vi "PAQmem_FindStartStopTimeIndex.vi"(8 "error in (no error)":errorcluster, 9 "End-time":timestamp, 10 "Start-time":timestamp, 11 "PAQ-memory in":refnum<class "PAQ-memory.lvclass">) -> (0 "error out":errorcluster, 1 "Size":i32, 2 "Start":i32, 3 "PAQ-memory out":refnum<class "PAQ-memory.lvclass">, 4 "time":timestamp[](array[timestamp]))   [LabVIEW 2020, in "Sgraph_lib_V1.lvlib" / "PAQ-memory.lvclass"]
doc: "Andre Koelewijn, 2 April 2021\n\nFind the index of the start and stop time when searching for a portion of the PAQ buffer section\nAdditional to the indexes this vi also delivers the time array of the searched data portion."
uses:
  PAQ-memory.lvclass
  PAQ-memory.lvclass/PAQ-memory.ctl
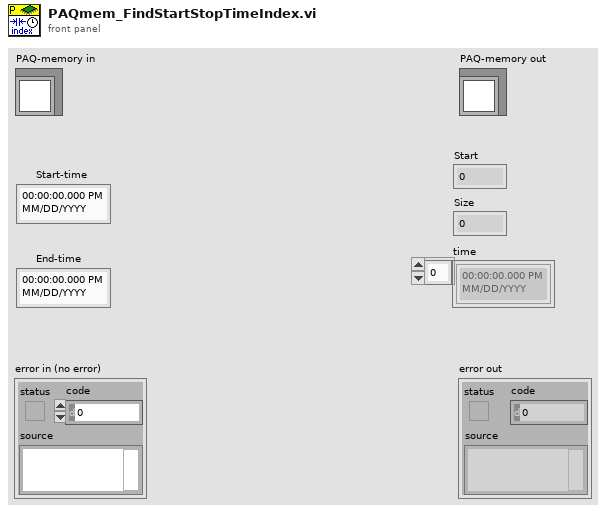
[diagram p1: front panel]
types:
  T1 = typedef "Sgraph_lib_V1.lvlib/FAMM.lvclass/typedef_PAQdata.ctl" = cluster{"TAGs":string[], "Time":refnum<data-value>, "TAGdata":cluster{"source":refnum<data-value>, "status":refnum<data-value>, "data":refnum<data-value>, "max":refnum<data-value>, "min":refnum<data-value>}[]}
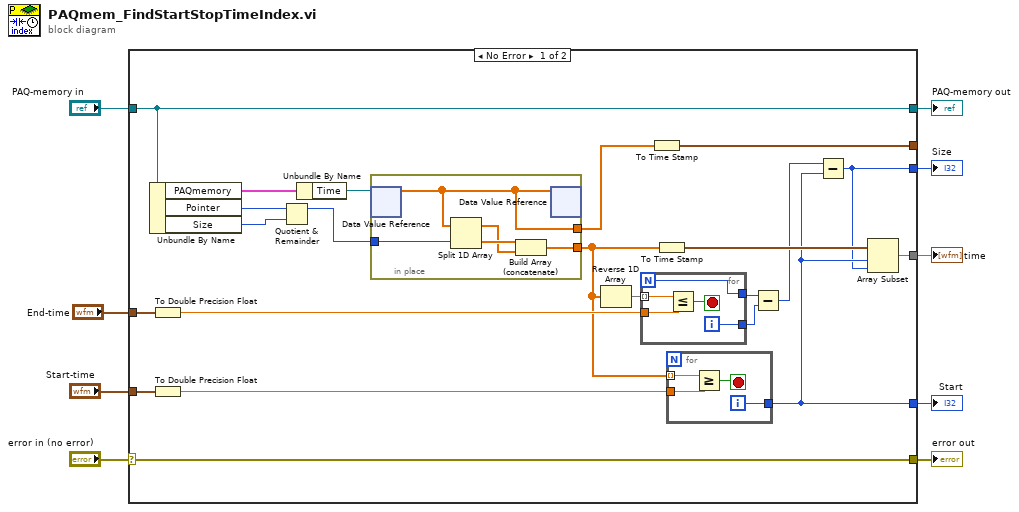
[diagram p0: block diagram]
diagram:
  n1 = case shown="No Error" "error in (no error)" {
    selector: "error in (no error)" -> [w31 w47]
    tunnel: [w31 w47] -> w8
    tunnel: [w29 w46] -> w6
    tunnel: "PAQ-memory in" -> [w29 w46]
    tunnel: [w23 _] -> w2
    tunnel: "Start-time" -> [w26 _]
    tunnel: [w19 _] -> w4
    tunnel: [w18 _] -> w3
    tunnel: "End-time" -> [w21 _]
    tunnel: [w10 _] -> _
    frame No Error {
      n2 = Unbundle By Name(w29) -> ("PAQmemory"=w30:T1, "Pointer"=w27:i32, "Size"=w22:i32)
      n3 = To Double Precision Float(number=w21) -> (double precision float=w20:dbl)
      n4 = To Double Precision Float(number=w26) -> (double precision float=w25:dbl)
      n5 = Quotient & Remainder(x=w27, y=w22) -> (x-y*floor(x/y)=w28:i32)  [unwired: 1 out]
      n6 = Unbundle By Name(w30) -> ("Time"=w12:refnum<data-value>)
      n7 = in-place {
        in-place-border: w28 -> [w45]
        in-place-border: [w42] -> w17
        in-place-border: [w41] -> w11
        n8 = in-place-dvr #1(w12) -> (w41:dbl[])  [unwired: 1 out]
        n9 = Split 1D Array(array=w41, index=w45) -> (first subarray=w43:dbl[], second subarray=w44:dbl[])
        n10 = Build Array (concatenate)(w44, w43) -> (w42:dbl[])
        n11 = in-place-dvr #1(w41) -> ()  [unwired: 2 out]
      }
      n12 = Reverse 1D Array(array=w17) -> (reversed array=w16:dbl[])
      n13 = for {
        N -> [w32]
        tunnel: w16 -> [w36] mode=indexing
        tunnel: w20 -> [w35]
        tunnel: [w33] -> w14
        tunnel: [w32] -> w15
        i -> [w33]
        stop <- w34 stop-if-true
        n14 = Less Or Equal?(x=w36, y=w35) -> (x <= y?=w34:bool)
      }
      n15 = To Time Stamp(1:w11) -> (0:w10:timestamp[])
      n16 = To Time Stamp(1:w17) -> (0:w24:timestamp[])
      n17 = for {
        tunnel: w17 -> [w40] mode=indexing
        tunnel: w25 -> [w39]
        tunnel: [w37] -> w19
        i -> [w37]
        stop <- w38 stop-if-true
        n18 = Greater Or Equal?(x=w40, y=w39) -> (x >= y?=w38:bool)
      }
      n19 = Subtract(x=w15, y=w14) -> (x-y=w13:i32)
      n20 = Subtract(x=w13, y=w19) -> (x-y=w18:i32)
      n21 = Array Subset(array=w24, index=w19, length=w18) -> (w23:timestamp[])
    }
    frame Error {
    }
  }
  "error out" <- w8
  "PAQ-memory out" <- w6
  "time" <- w2
  "Start" <- w4
  "Size" <- w3
